vi "Laser ops tester.vi"() -> ()   [LabVIEW 2017]
uses:
  Serial Comms/Visa resource.ctl
  Laser Ops (Generic)/Type Defs/Ls1 Operations.ctl
panel:
  in  "stop":bool
  in  "PreChrp1 \nVisa resource":T1
  in  "Ls1 Visa \nresource":T1
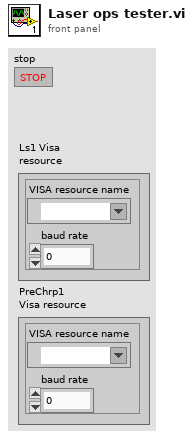
[diagram p1: front panel]
types:
  T1 = typedef "Visa resource.ctl" = cluster{"VISA resource name":refnum<visa-resource-name>, "baud rate":u32}
  T2 = typedef "Ls1 Operations.ctl" = enum16{"Initialise Connections", "Initialise system", "Check Status", "Open/Close Shutter", "Start/Stop Pump Peak Hold", "Set wavelength", "Close"}
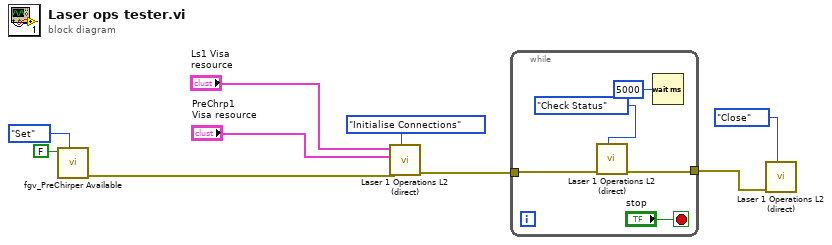
[diagram p0: block diagram]
diagram:
  n1 = call "fgv_PreChirper Available.vi"("FGV Actions"=enum16{"Get", "Set"}."Set", "PreChirper Available ? IN"=FALSE) -> ("error out"=w4:errorcluster)  [unwired: 8 in, 1 out]
  n2 = call "Laser 1 Operations L2 (direct).vi"("Laser Ops\n actions"=Ls1_Operations."Initialise Connections" ("Laser Ops\n actions"), "error in (no error)"=w4, "PreChrp1 \nVisa resource"="PreChrp1 \nVisa resource", "Ls1 Visa \nresource"="Ls1 Visa \nresource") -> ("error out"=w3:errorcluster)  [unwired: 3 in, 4 out]
  n3 = while {
    tunnel: w3 -> [w14]
    tunnel: [w13] -> w2
    stop <- "stop" stop-if-true
    n4 = call "Laser 1 Operations L2 (direct).vi"("Laser Ops\n actions"=Ls1_Operations."Check Status" ("Laser Ops\n actions"), "error in (no error)"=w14) -> ("error out"=w13:errorcluster)  [unwired: 5 in, 4 out]
    n5 = Wait (ms)(milliseconds to wait=u32 5000) -> ()  [unwired: 1 out]
  }
  n6 = call "Laser 1 Operations L2 (direct).vi"("Laser Ops\n actions"=Ls1_Operations."Close" ("Laser Ops\n actions"), "error in (no error)"=w2) -> ()  [unwired: 5 in, 5 out]
